vi "Start Idle Processes if Running.vi"(8 "error in (no error)":errorcluster, 10 "Rig Process":refnum<class "Process.lvclass">, 11 "Rig in":refnum<class "Application.lvclass">) -> (0 "error out":errorcluster, 2 "Rig Process Out":refnum<class "Process.lvclass">, 3 "Rig out":refnum<class "Application.lvclass">)   [LabVIEW 2020, in "Application.lvclass"]
uses:
  Application.lvclass
  Process/Process.lvclass
  Application.lvclass/Application.ctl
  Process/Process.lvclass/Process.ctl
  <vilib>/Utility/error.llb/Clear Errors.vi
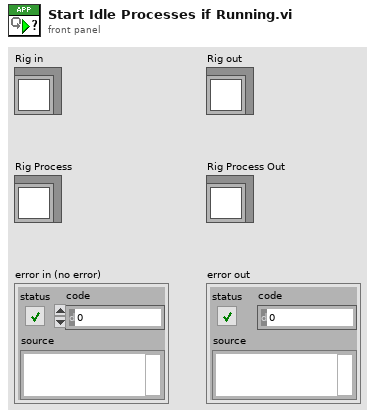
[diagram p1: front panel]
types:
  T1 = typedef "Process.lvclass/Lifecycle State.ctl" = enum16{"Uninitialized", "Initialized", "Started", "Running", "Stopped", "Finished"}
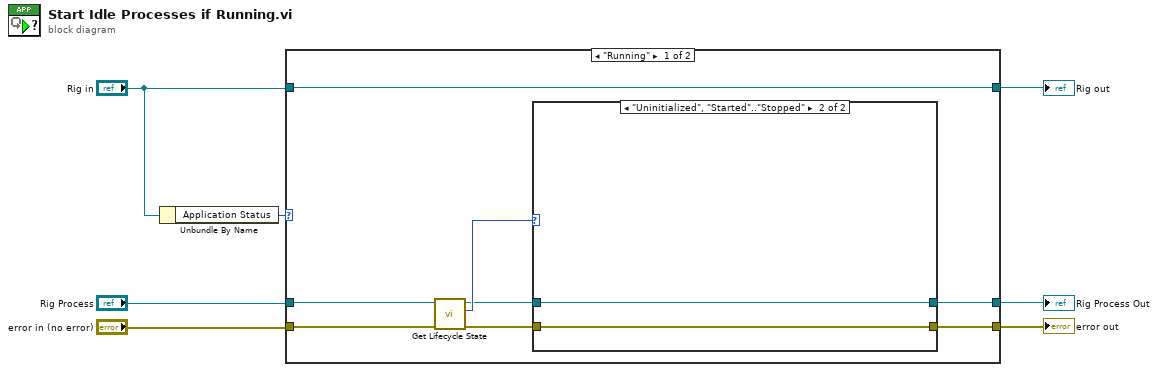
[diagram p0: block diagram]
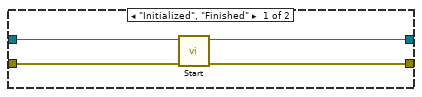
[diagram p2: hidden frame]
diagram:
  n1 = Unbundle By Name("Rig in") -> ("Application Status"=w1:enum16{"Idle", "Running"})
  n2 = case shown="\"Running\"" w1 {
    tunnel: "Rig in" -> [w15 w23]
    tunnel: [w8 w24] -> w6
    tunnel: [w9 w22] -> w7
    tunnel: [w15 w23] -> w5
    tunnel: "Rig Process" -> [w14 w24]
    tunnel: "error in (no error)" -> [w13 w22]
    frame "Running" {
      n3 = call "Get Lifecycle State.vi"("error in (no error)"=w13, "Process In"=w14) -> ("error out"=w10:errorcluster, "Lifecycle State"=w12:T1, "Process Out"=w11:refnum<class "Process.lvclass">)  [unwired: 6 in, 1 out]
      n4 = case shown="\"Uninitialized\", \"Started\"..\"Stopped\"" w12 {
        tunnel: w11 -> [w19 w21]
        tunnel: w10 -> [w18 w20]
        tunnel: [w17 w20] -> w9
        tunnel: [w16 w21] -> w8
        frame "Initialized", "Finished" {
          n5 = call "Start.vi"("error in (no error)"=w18, "Process In"=w19) -> ("error out"=w17:errorcluster, "Process Out"=w16:refnum<class "Process.lvclass">)  [unwired: 8 in]
        }
        frame "Uninitialized", "Started".."Stopped" {
        }
      }
    }
    frame "Idle" {
    }
  }
  "error out" <- w7
  "Rig Process Out" <- w6
  "Rig out" <- w5
